vi "_Check Limit.vi"(4 "Header":string="Starting:", 5 "Min (0)":dbl, 6 "Current":dbl, 7 "Max (100)":dbl=100.0) -> (1 "Max Reached":bool, 3 "ProgressBar":string)   [LabVIEW 2015]
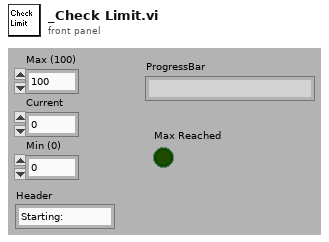
[diagram p1: front panel]
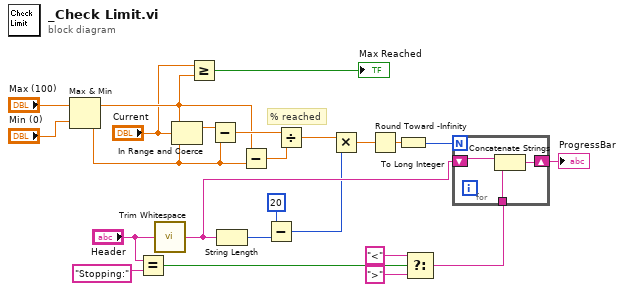
[diagram p0: block diagram]
diagram:
  # "% reached"
  n1 = Max & Min(x="Max (100)", y="Min (0)") -> (max(x,y)=w13:dbl, min(x,y)=w18:dbl)
  n2 = Equal?(x="Header", y="Stopping:" ("Header (10Ch)")) -> (x = y?=w4:bool)
  n3 = call <vilib>:"Trim Whitespace.vi"("string"="Header") -> ("trimmed string"=w10:string)  [unwired: 1 in]
  n4 = In Range and Coerce(upper limit=w13, x="Current", lower limit=w18) -> (coerced(x)=w19:dbl)  [unwired: 1 out]
  n5 = Greater Or Equal?(x="Current", y=w13) -> (x >= y?=→"Max Reached":bool)
  n6 = Subtract(x=w19, y=w18) -> (x-y=w17:dbl)
  n7 = String Length(string=w10) -> (length=w9:i32)
  n8 = Subtract(x=w13, y=w18) -> (x-y=w21:dbl)
  n9 = Subtract(x=20, y=w9) -> (x-y=w7:i32)
  n10 = Divide(x=w17, y=w21) -> (x/y=w20:dbl)
  n11 = Multiply(x=w20, y=w7) -> (x*y=w16:dbl)
  n12 = Round Toward -Infinity(1:w16) -> (0:w14:dbl)
  n13 = To Long Integer(number=w14) -> (32bit integer=w15:i32)
  n14 = Select(t="<" ("string"), s=w4, f=">" ("string")) -> (s? t:f=w1:string)
  n15 = for {
    N: w15 -> [_]
    shift-right: [w26] -> w24
    shift-left: w10 -> [w27]
    tunnel: w1 -> [w25]
    n16 = Concatenate Strings(w27, w25) -> (w26:string)
  }
  "ProgressBar" <- w24
